vi "Producer Consumer Events.vi"() -> ()   [LabVIEW 2017]
doc: "Use this template to build a producer/consumer design pattern with events to produce queue items. Use this design pattern instead of the User Interface Event Handler pattern for user interfaces when you want to execute code asynchronously in response to an event without slowing the user interface responsiveness."
uses:
  <vilib>/Waveform/WDTOps.llb/WDT Index Channel DBL.vi
panel:
  in  "Sekvence":T1(ring)
  out "Signali":dynamicdata(graph) caption="data"
  in  "Start/Pause":bool
  out "?":dbl format="%#5_3g"
  out "3":bool
  out "2":bool
  out "1":bool
  in  "output cluster":cluster{"data":dynamicdata, "Numeric":dbl}
  out "Sekvenca":dbl[](array[numeric])
  in  "No. Samples":i16=1900 min=500 max=1900 step=100
  in  "Enqueue Element":bool
  in  "stop":bool
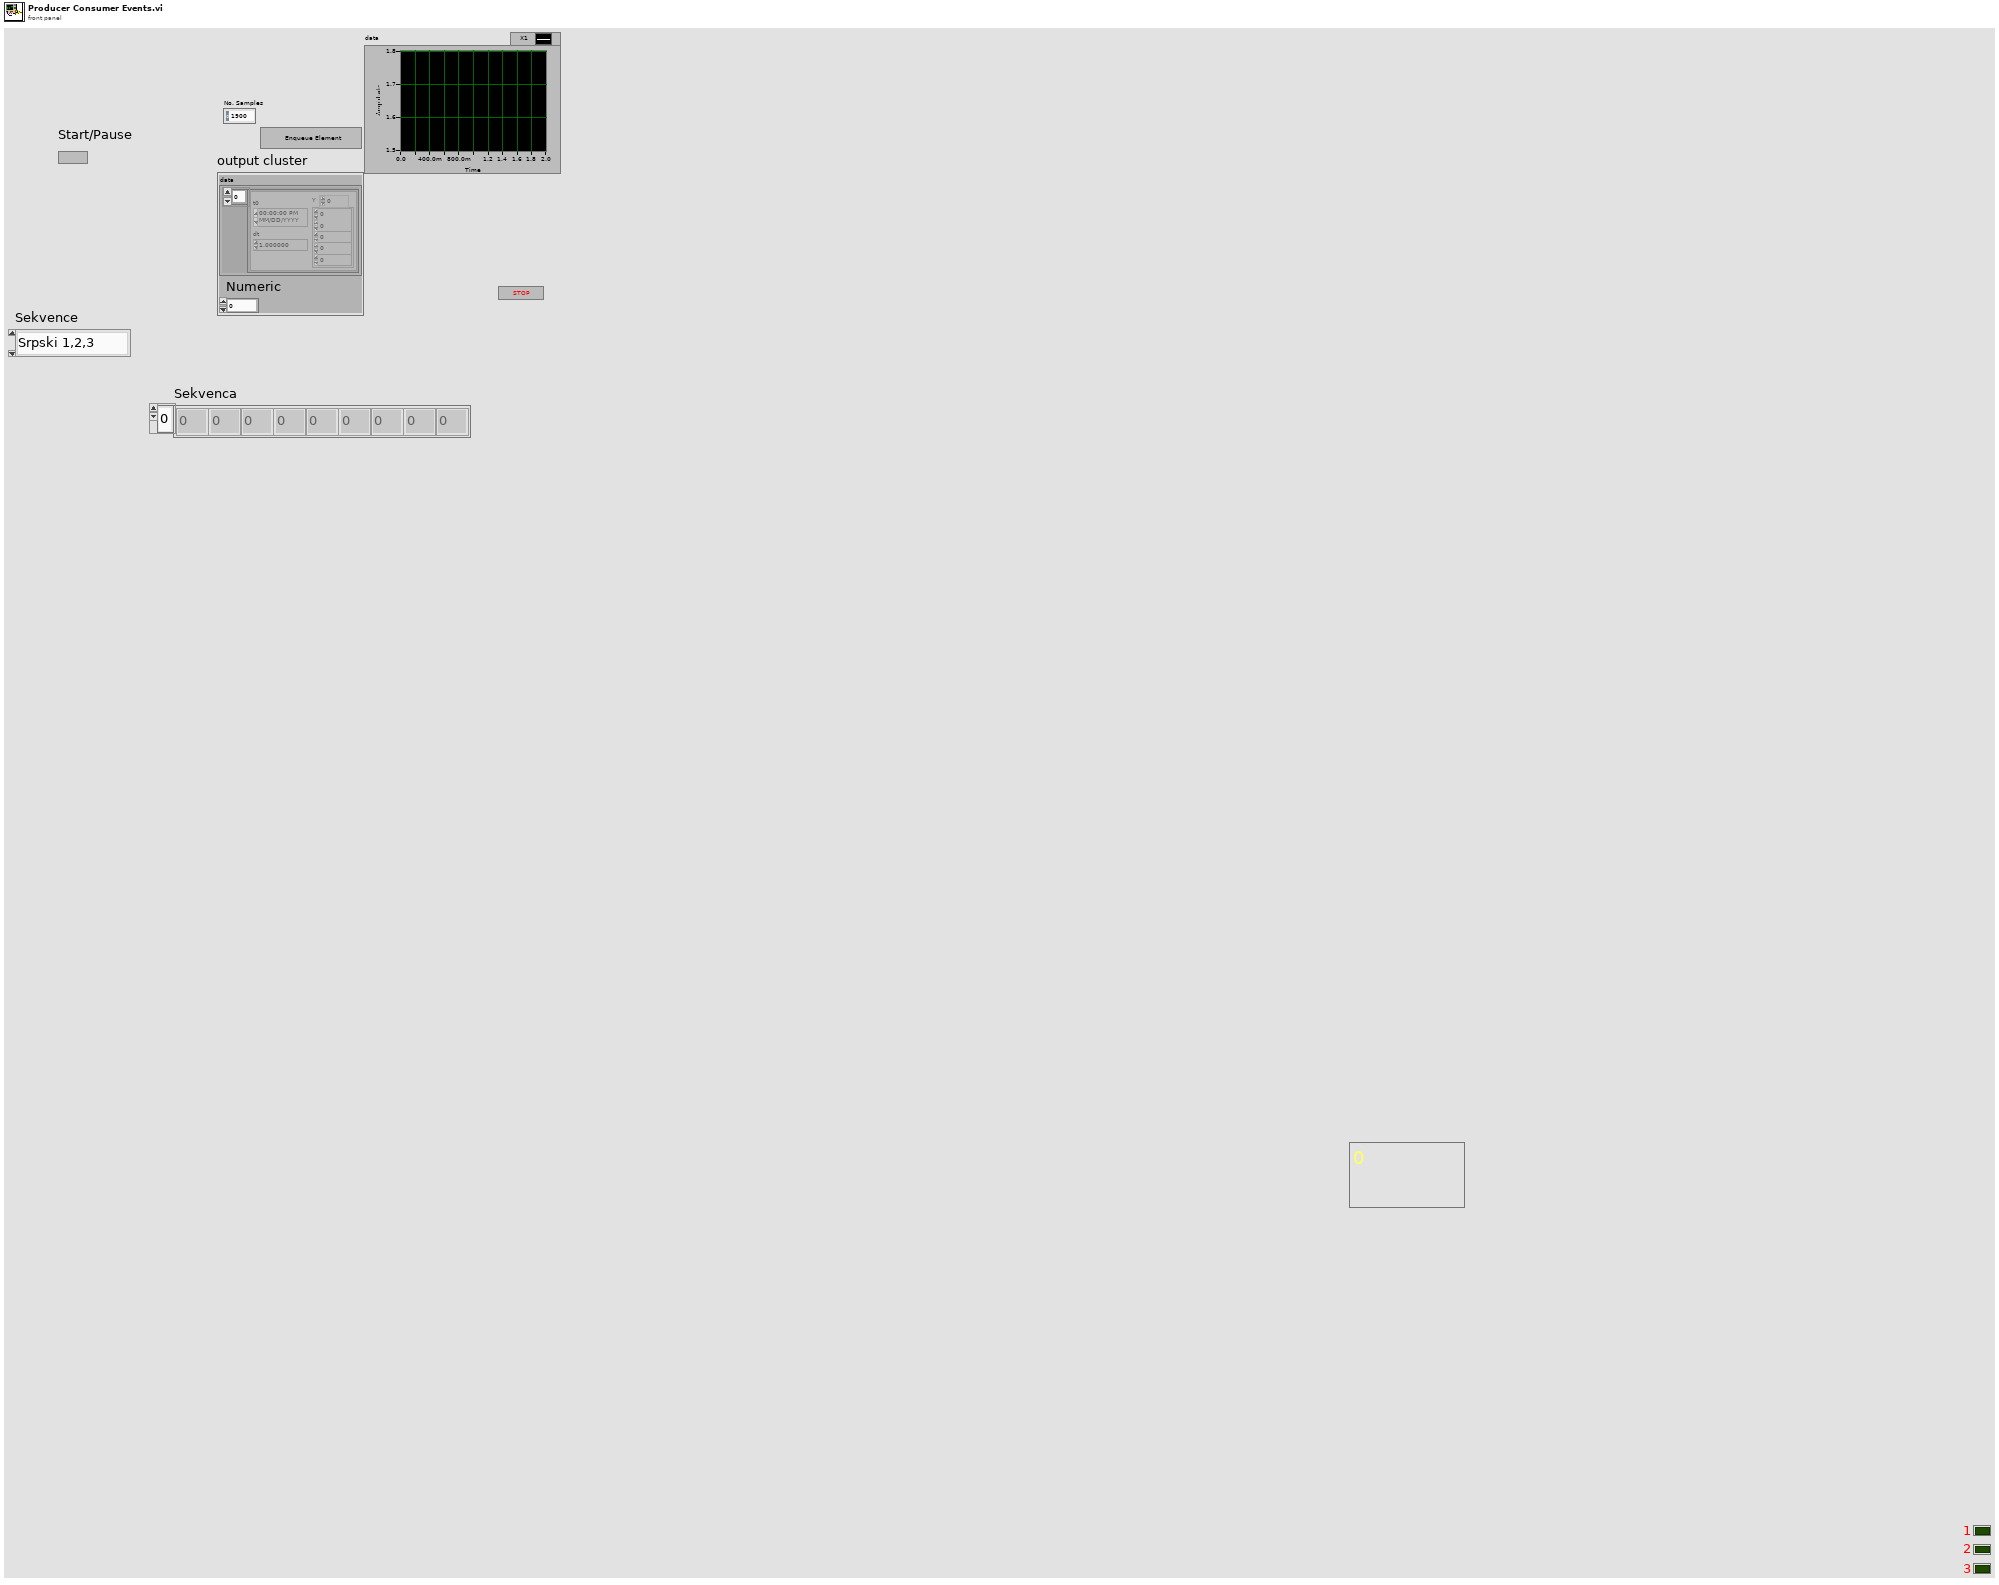
[diagram p1: front panel]
types:
  T1 = enum16{"Srpski 1,2,3", "Engleski 1,2,3", "Kombinacije"}
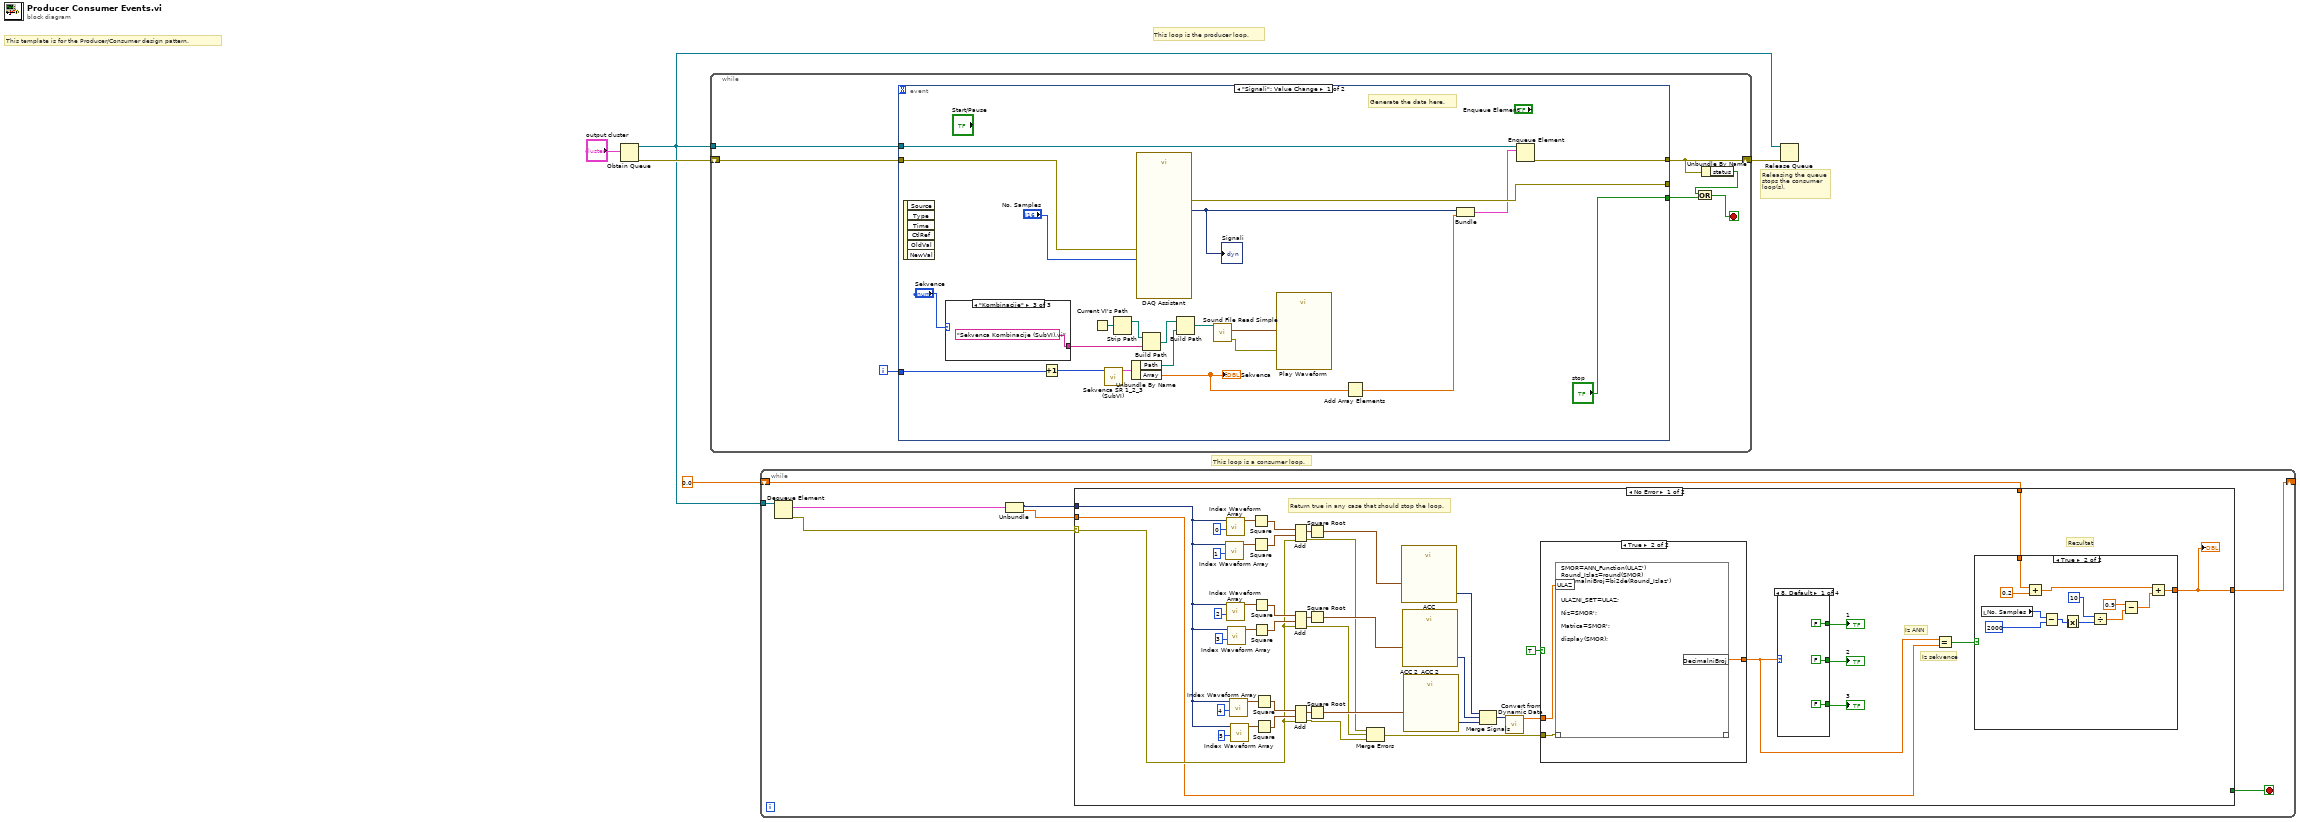
[diagram p0: block diagram]
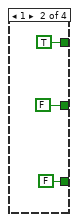
[diagram p3: hidden frame]
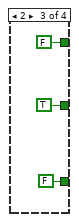
[diagram p4: hidden frame]
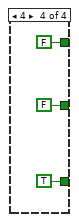
[diagram p5: hidden frame]
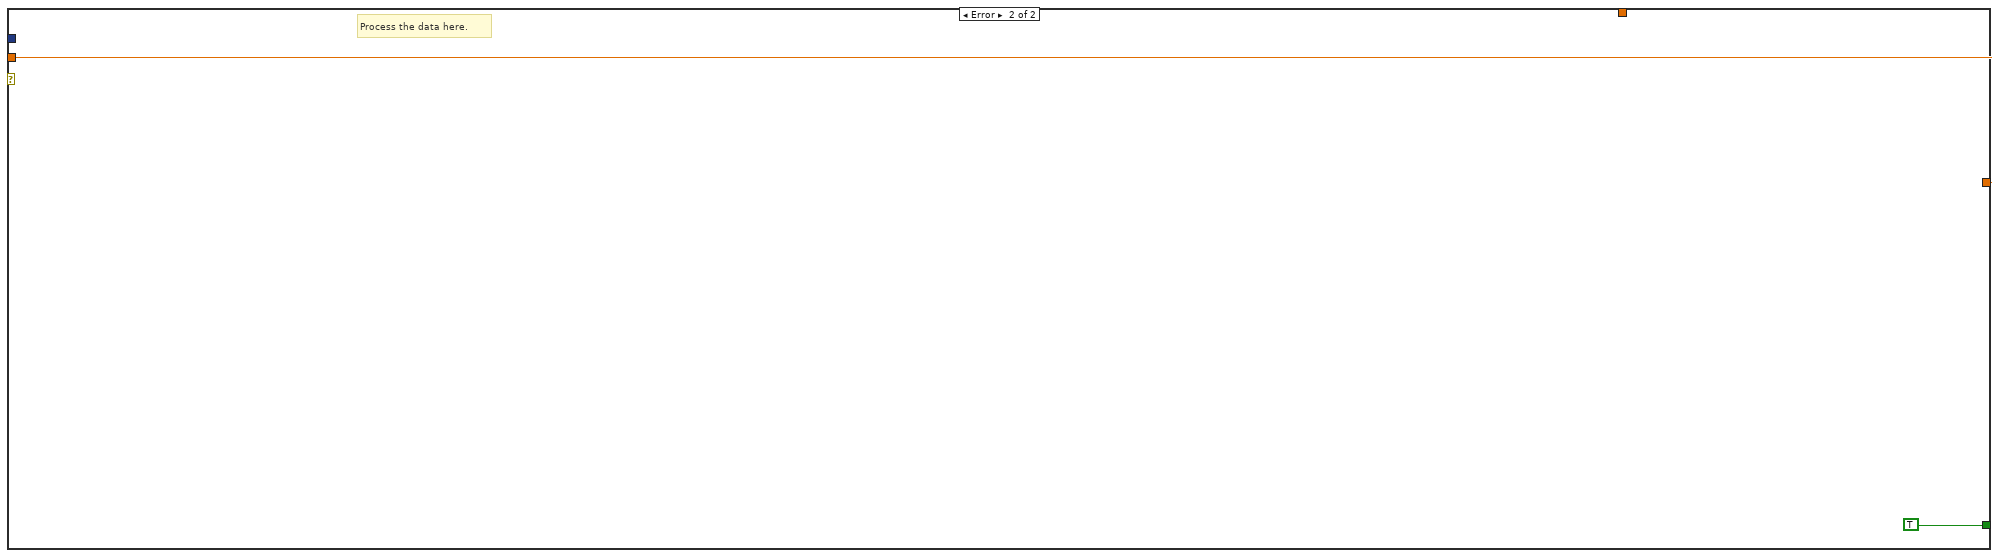
[diagram p7: hidden frame]
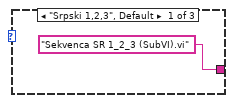
[diagram p8: hidden frame]
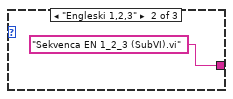
[diagram p9: hidden frame]
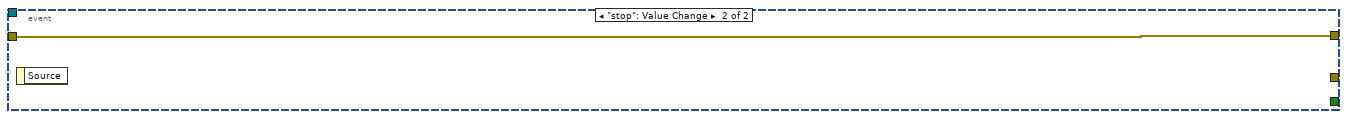
[diagram p10: hidden frame]
diagram:
  # "This loop is a consumer loop."
  # "This loop is the producer loop."
  # "Releasing the queue stops the consumer loop(s)."
  # "This template is for the Producer/Consumer design pattern."
  n1 = Obtain Queue(element data type="output cluster") -> (queue out=w3:refnum<queue>, error out=w5:errorcluster)  [unwired: 4 in, 1 out]
  n2 = while {
    shift-right: [w9] -> w4
    shift-left: w5 -> [w11]
    tunnel: w3 -> [w12]
    i -> [w10]
    stop <- w7 stop-if-true
    n3 = event shown="[0] \"Signali\": Value Change" {
      selector: _ -> [_ _]
      dyn-events: _ -> [_ _]
      timeout: _ -> [_ _]
      tunnel: w12 -> [w34 _]
      tunnel: w11 -> [w31 w38]
      tunnel: [w33 w38] -> w9
      tunnel: [w30 _] -> _
      tunnel: w10 -> [w23 _]
      tunnel: ["stop" _] -> w6
      event "Signali": Value Change {
        # "Generate the data here."
        n4 = event-data() -> ()  [unwired: 1 in, 6 out]
        n5 = case shown="\"Kombinacije\"" "Sekvence" {
          tunnel: ["Sekvenca SR 1_2_3 (SubVI).vi" "Sekvenca EN 1_2_3 (SubVI).vi" "Sekvenca Kombinacije (SubVI).vi"] -> w13
          frame "Srpski 1,2,3", Default {
          }
          frame "Engleski 1,2,3" {
          }
          frame "Kombinacije" {
          }
        }
        n6 = Increment(x=w23) -> (x+1=w15:i32)
        n7 = Current VI's Path() -> (path=w20:path)
        n8 = call "Sekvenca SR 1_2_3 (SubVI).vi"("Ulaz"=w15) -> ("Cluster 41"=w16:cluster{"Path":path, "Array":dbl[]})  [unwired: 9 in, 1 out]
        n9 = Strip Path(path=w20) -> (stripped path=w18:path)  [unwired: 1 out]
        n10 = Unbundle By Name(w16) -> ("Path"=w17:path, "Array"=w21:dbl[])
        "Sekvenca" <- w21
        n11 = call "DAQ Assistant"("number of samples"="No. Samples", "error in"=w31) -> ("data"=w29:dynamicdata, "error out"=w30:errorcluster)  [unwired: 14 in, 2 out]
        "Signali" <- w29
        n12 = Build Path(base path=w18, name or relative path=w13) -> (appended path=w19:path)
        n13 = Build Path(base path=w19, name or relative path=w17) -> (appended path=w27:path)
        n14 = call <vilib>:"Sound File Read Simple.vi"("path"=w27) -> ("error out"=w28:errorcluster, "data"=w26:waveform(dbl)[])  [unwired: 7 in, 2 out]
        n15 = call "Play Waveform"("Data"=w26, "error in"=w28) -> ()  [unwired: 17 in, 1 out]
        n16 = Add Array Elements(numeric array=w21) -> (sum=w25:dbl)
        n17 = Bundle("data"=w29, "Numeric"=w25) -> (w24:cluster{"data":dynamicdata, "Numeric":dbl})  [unwired: 1 in]
        n18 = Enqueue Element(queue=w34, element=w24) -> (error out=w33:errorcluster)  [unwired: 2 in, 2 out]
      }
      event "stop": Value Change {
        n19 = event-data() -> ()  [unwired: 1 in, 1 out]
      }
    }
    n20 = Unbundle By Name(w9) -> ("status"=w8:bool)
    n21 = Or(x=w8, y=w6) -> (x .or. y?=w7:bool)
  }
  n22 = while {
    tunnel: w3 -> [w46]
    shift-right: [w40] -> _
    shift-left: 0.0 -> [w41]
    stop <- w39 stop-if-true
    n23 = Dequeue Element(queue=w46) -> (element=w44:cluster{"data":dynamicdata, "Numeric":dbl}, error out=w45:errorcluster)  [unwired: 2 in, 2 out]
    n24 = Unbundle(w44) -> ("data"=w43:dynamicdata, "Numeric"=w42:dbl)
    n25 = case shown="No Error" w45 {
      selector: w45 -> [w59 _]
      tunnel: [w51 w119] -> w40
      tunnel: w43 -> [w49 _]
      tunnel: w42 -> [w48 w119]
      tunnel: w41 -> [w47 _]
      tunnel: [_ TRUE] -> w39
      frame No Error {
        # "Rezultat"
        # "Iz sekvence"
        # "Iz ANN"
        # "Return true in any case that should stop the loop."
        n26 = call-poly <vilib>:"Index Waveform Array.vi"("index"=1, "waveform array"=w49) -> ("waveform"=w68:waveform(dbl))  [unwired: 8 in, 1 out]
        n27 = call-poly <vilib>:"Index Waveform Array.vi"("index"=0, "waveform array"=w49) -> ("waveform"=w67:waveform(dbl))  [unwired: 8 in, 1 out]
        n28 = call-poly <vilib>:"Index Waveform Array.vi"("index"=2, "waveform array"=w49) -> ("waveform"=w69:waveform(dbl))  [unwired: 8 in, 1 out]
        n29 = call-poly <vilib>:"Index Waveform Array.vi"("index"=3, "waveform array"=w49) -> ("waveform"=w70:waveform(dbl))  [unwired: 8 in, 1 out]
        n30 = call-poly <vilib>:"Index Waveform Array.vi"("index"=4, "waveform array"=w49) -> ("waveform"=w71:waveform(dbl))  [unwired: 8 in, 1 out]
        n31 = call-poly <vilib>:"Index Waveform Array.vi"("index"=5, "waveform array"=w49) -> ("waveform"=w72:waveform(dbl))  [unwired: 8 in, 1 out]
        n32 = Square(x=w67) -> (x^2=w73:waveform(dbl))
        n33 = Square(x=w68) -> (x^2=w74:waveform(dbl))
        n34 = Square(x=w69) -> (x^2=w75:waveform(dbl))
        n35 = Square(x=w70) -> (x^2=w76:waveform(dbl))
        n36 = Square(x=w71) -> (x^2=w77:waveform(dbl))
        n37 = Square(x=w72) -> (x^2=w78:waveform(dbl))
        n38 = Add(1:w74, 2:w73, 4:w59) -> (0:w79:waveform(dbl), 3:w82:errorcluster)
        n39 = Add(1:w76, 2:w75, 4:w59) -> (0:w80:waveform(dbl), 3:w83:errorcluster)
        n40 = Add(1:w78, 2:w77, 4:w59) -> (0:w81:waveform(dbl), 3:w84:errorcluster)
        n41 = Square Root(x=w79) -> (sqrt(x)=w87:waveform(dbl))
        n42 = Square Root(x=w80) -> (sqrt(x)=w88:waveform(dbl))
        n43 = Square Root(x=w81) -> (sqrt(x)=w89:waveform(dbl))
        n44 = Merge Errors(w82, w83, w84) -> (w58:errorcluster)
        n45 = call "ACC"("Signals"=w87) -> ("Peak to Peak"=w90:dynamicdata)  [unwired: 13 in, 1 out]
        n46 = call "ACC 2"("Signals"=w88) -> ("Peak to Peak"=w85:dynamicdata)  [unwired: 13 in, 1 out]
        n47 = call "ACC 2"("Signals"=w89) -> ("Peak to Peak"=w86:dynamicdata)  [unwired: 13 in, 1 out]
        n48 = Merge Signals(w90, w85, w86) -> (w60:dynamicdata)
        n49 = call "Convert from Dynamic Data"("Dynamic Data Type"=w60) -> ("Array"=w56:dbl[])  [unwired: 3 in]
        n50 = case shown="True" TRUE {
          tunnel: [_ w117] -> w50
          tunnel: w58 -> [_ w116]
          tunnel: w56 -> [_ w115]
          frame False {
          }
          frame True {
            n51 = script code="SMOR=ANN_Function(ULAZ')\nRound_Izlaz=round(SMOR)\nDecimalniBroj=bi2de(Round_Izlaz')\n\n\nULAZNI_SET=ULAZ;\n\nNiz=SMOR';\n\nMatrica=SMOR';\n\ndisplay(SMOR);"("??"=w116, "ULAZ"=w115) -> ("DecimalniBroj"=w117:dbl)  [unwired: 1 out]
          }
        }
        n52 = case shown="8, Default" w50 {
          tunnel: [FALSE ("DOLE") FALSE ("DOLE") FALSE ("DOLE") TRUE ("DOLE")] -> w53
          tunnel: [FALSE ("SREDINA") FALSE ("SREDINA") TRUE ("SREDINA") FALSE ("SREDINA")] -> w54
          tunnel: [FALSE ("GORE") TRUE ("GORE") FALSE ("GORE") FALSE ("GORE")] -> w55
          frame 8, Default {
          }
          frame 1 {
          }
          frame 2 {
          }
          frame 4 {
          }
        }
        "1" <- w55
        "2" <- w54
        "3" <- w53
        n53 = Equal?(x=w50, y=w48) -> (x = y?=w52:bool)
        n54 = case shown="True" w52 {
          tunnel: [_ w92] -> w51
          tunnel: w47 -> [_ w91]
          frame False {
          }
          frame True {
            n55 = local read "No. Samples"() -> (w100:i16)
            n56 = Add(x=w91, y=0.2) -> (x+y=w97:dbl)
            n57 = Subtract(x=w100, y=2000) -> (x-y=w102:i32)
            n58 = Absolute Value(x=w102) -> (abs(x)=w101:i32)
            n59 = Divide(x=10, y=w101) -> (x/y=w99:dbl)
            n60 = Subtract(x=0.9, y=w99) -> (x-y=w98:dbl)
            n61 = Add(x=w97, y=w98) -> (x+y=w92:dbl)
          }
        }
        "?" <- w51
      }
      frame Error {
        # "Process the data here."
      }
    }
  }
  n62 = Release Queue(queue=w3, error in (no error)=w4) -> ()  [unwired: 1 in, 3 out]
